vi "Config Digital Output.vi"(0 "VISA resource name":refnum<visa-resource-name>, 7 "Digital Output (0)":dbl min=0.0 max=31.0 step=1.0, 11 "error in (no error)":errorcluster) -> (4 "VISA resource name out":refnum<visa-resource-name>, 15 "error out":errorcluster)   [LabVIEW 2024, in "Lake Shore Cryotronics 370.lvlib"]
doc: "This VI specifies the manual digital output settings using bit weighting. This function is only active if no Model 3716 Scanner is installed."
uses:
  Lake Shore Cryotronics 370.lvlib
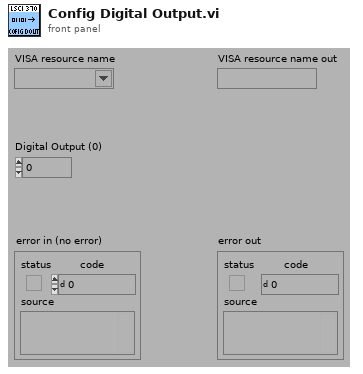
[diagram p1: front panel]
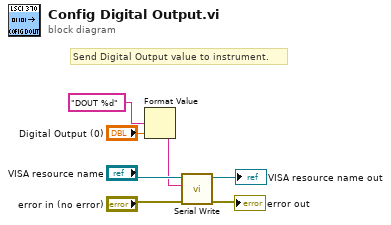
[diagram p0: block diagram]
diagram:
  # "Send Digital Output value to instrument."
  n1 = Format Value(format string="DOUT %d", value (0)="Digital Output (0)") -> (output string=w1:string)  [unwired: 1 in]
  n2 = call "Serial Write.vi"("error in (no error)"="error in (no error)", "Write Buffer (\"\")"=w1, "VISA resource name"="VISA resource name") -> ("error out"=→"error out":errorcluster, "VISA resource name out"=→"VISA resource name out":refnum<visa-resource-name>)  [unwired: 6 in, 1 out]
